vi "ConfigMeasData.vi"(8 "error in (no error)":errorcluster, 10 "ColumnName":string[](array[string]), 11 "DUTMotor in":refnum<class "DUTMotor.lvclass">) -> (0 "error out":errorcluster, 3 "DUTMotor out":refnum<class "DUTMotor.lvclass">)   [LabVIEW 2024, in "DUTMotor Actor.lvlib" / "DUTMotor.lvclass"]
uses:
  DUTMotor.lvclass
  DUTMotor.lvclass/DUTMotor.ctl
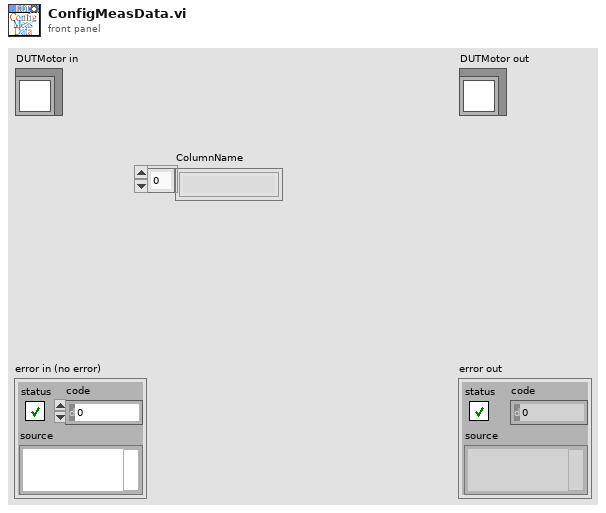
[diagram p1: front panel]
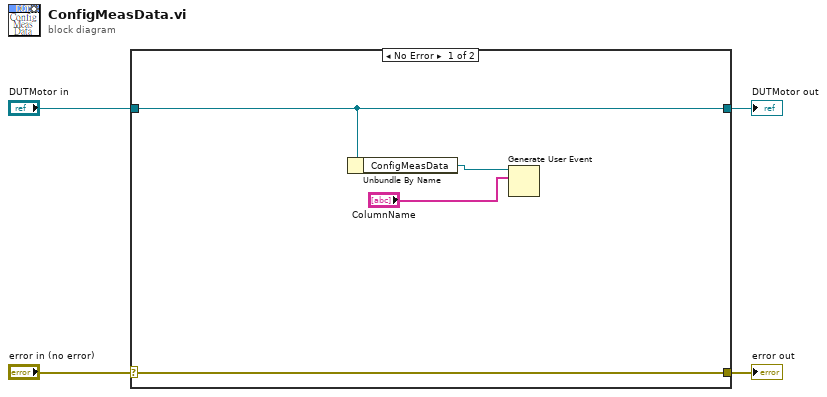
[diagram p0: block diagram]
diagram:
  n1 = case shown="No Error" "error in (no error)" {
    selector: "error in (no error)" -> [w8 w10]
    tunnel: [w8 w10] -> w3
    tunnel: [w7 w9] -> w1
    tunnel: "DUTMotor in" -> [w7 w9]
    frame No Error {
      n2 = Unbundle By Name(w7) -> ("ConfigMeasData"=w6:refnum<user-event>)
      n3 = Generate User Event(user event=w6, event data cluster="ColumnName") -> ()  [unwired: 2 in, 2 out]
    }
    frame Error {
    }
  }
  "error out" <- w3
  "DUTMotor out" <- w1
